vi "LJM_LoadConstants.vi"   [LabVIEW 2020]
uses:
  LabJackM.framework
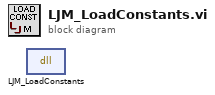
[diagram p0: block diagram]
diagram:
  n1 = dll-call lib="LabJackM.framework" fn="LJM_LoadConstants"() -> ()  [unwired: 4 in, 2 out]
